vi "9235_9236_9237 4Ch Analog Input.vi"(1 "9235/9236/9237 I/O":T1={"9235/9236/9237 AI0"="NI 9235/AI0", "9235/9236/9237 AI1"="NI 9235/AI1", "9235/9236/9237 AI2"="NI 9235/AI2", "9235/9236/9237 AI3"="NI 9235/AI3"}) -> (0 "Packets":u64[](array[numeric]))   [LabVIEW 2010]
uses:
  <vilib>/eio/EIONode/EIONode.xnode
  <vilib>/rvi/eio/nirviEIOImplementation/nirviEIOImplementation.xnode
  <vilib>/rvi/eio/common/nirviEmuClasses.ctl
  <vilib>/rvi/eio/common/nirviEmuTemplateMethod_noerrors.vi
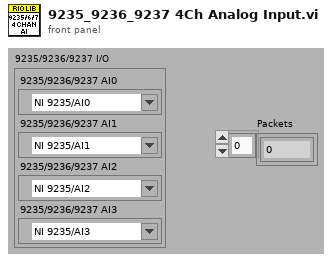
[diagram p1: front panel]
types:
  T1 = cluster{"9235/9236/9237 AI0":refnum<k21>, "9235/9236/9237 AI1":refnum<k21>, "9235/9236/9237 AI2":refnum<k21>, "9235/9236/9237 AI3":refnum<k21>}
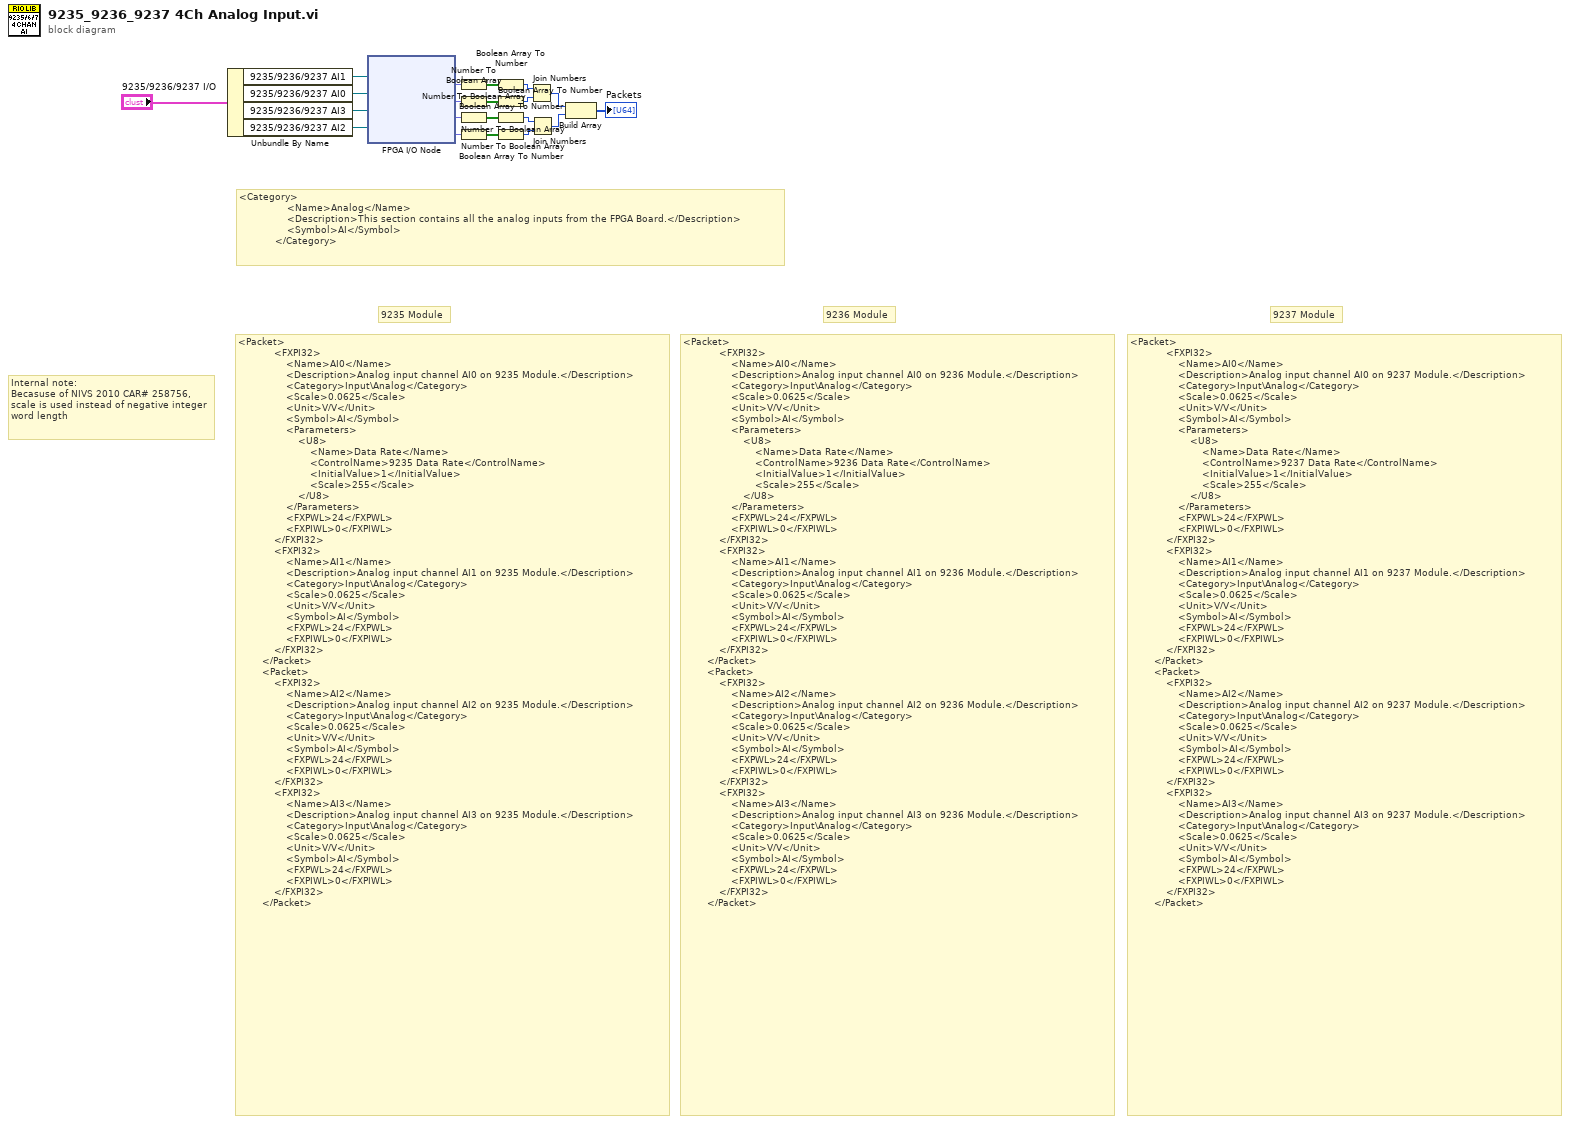
[diagram p0: block diagram]
diagram:
  # "9237 Module"
  # "<Packet>\n            <FXPI32>\n                <Name>AI0</Name>\n                <Description>Analog input channel AI0 on 9237 Module.</Description>\n                <Category>Input\\Analog</Category>\n                <Scale>0.0625</Scale>\n                <Unit>V/V</Unit>\n                <Symbol>AI</Symbol>\n                <Parameters>\n                    <U8>\n                        <Name>Data Rate</Name>\n                        <ControlName>9237 Data Rate</ControlName>\n                        <InitialValue>1</InitialValue>\n                        <Scale>255</Scale>\n                    </U8>\n                </Parameters>\n                <FXPWL>24</FXPWL>\n                <FXPIWL>0</FXPIWL>\n            </FXPI32>\n            <FXPI32>\n                <Name>AI1</Name>\n                <Description>Analog input channel AI1 on 9237 Module.</Description>\n                <Category>Input\\Analog</Category>\n                <Scale>0.0625</Scale>\n                <Unit>V/V</Unit>\n                <Symbol>AI</Symbol>\n                <FXPWL>24</FXPWL>\n                <FXPIWL>0</FXPIWL>\n            </FXPI32>\n        </Packet>\n        <Packet>\n            <FXPI32>\n                <Name>AI2</Name>\n                <Description>Analog input channel AI2 on 9237 Module.</Description>\n                <Category>Input\\Analog</Category>\n                <Scale>0.0625</Scale>\n                <Unit>V/V</Unit>\n                <Symbol>AI</Symbol>\n                <FXPWL>24</FXPWL>\n                <FXPIWL>0</FXPIWL>\n            </FXPI32>\n            <FXPI32>\n                <Name>AI3</Name>\n                <Description>Analog input channel AI3 on 9237 Module.</Description>\n                <Category>Input\\Analog</Category>\n                <Scale>0.0625</Scale>\n                <Unit>V/V</Unit>\n                <Symbol>AI</Symbol>\n                <FXPWL>24</FXPWL>\n                <FXPIWL>0</FXPIWL>\n            </FXPI32>\n        </Packet>"
  # "9236 Module"
  # "<Packet>\n            <FXPI32>\n                <Name>AI0</Name>\n                <Description>Analog input channel AI0 on 9236 Module.</Description>\n                <Category>Input\\Analog</Category>\n                <Scale>0.0625</Scale>\n                <Unit>V/V</Unit>\n                <Symbol>AI</Symbol>\n                <Parameters>\n                    <U8>\n                        <Name>Data Rate</Name>\n                        <ControlName>9236 Data Rate</ControlName>\n                        <InitialValue>1</InitialValue>\n                        <Scale>255</Scale>\n                    </U8>\n                </Parameters>\n                <FXPWL>24</FXPWL>\n                <FXPIWL>0</FXPIWL>\n            </FXPI32>\n            <FXPI32>\n                <Name>AI1</Name>\n                <Description>Analog input channel AI1 on 9236 Module.</Description>\n                <Category>Input\\Analog</Category>\n                <Scale>0.0625</Scale>\n                <Unit>V/V</Unit>\n                <Symbol>AI</Symbol>\n                <FXPWL>24</FXPWL>\n                <FXPIWL>0</FXPIWL>\n            </FXPI32>\n        </Packet>\n        <Packet>\n            <FXPI32>\n                <Name>AI2</Name>\n                <Description>Analog input channel AI2 on 9236 Module.</Description>\n                <Category>Input\\Analog</Category>\n                <Scale>0.0625</Scale>\n                <Unit>V/V</Unit>\n                <Symbol>AI</Symbol>\n                <FXPWL>24</FXPWL>\n                <FXPIWL>0</FXPIWL>\n            </FXPI32>\n            <FXPI32>\n                <Name>AI3</Name>\n                <Description>Analog input channel AI3 on 9236 Module.</Description>\n                <Category>Input\\Analog</Category>\n                <Scale>0.0625</Scale>\n                <Unit>V/V</Unit>\n                <Symbol>AI</Symbol>\n                <FXPWL>24</FXPWL>\n                <FXPIWL>0</FXPIWL>\n            </FXPI32>\n        </Packet>"
  # "Internal note:\nBecasuse of NIVS 2010 CAR# 258756, scale is used instead of negative integer word length"
  # "9235 Module"
  # "<Category>\n                <Name>Analog</Name>\n                <Description>This section contains all the analog inputs from the FPGA Board.</Description>\n                <Symbol>AI</Symbol>\n            </Category>"
  # "<Packet>\n            <FXPI32>\n                <Name>AI0</Name>\n                <Description>Analog input channel AI0 on 9235 Module.</Description>\n                <Category>Input\\Analog</Category>\n                <Scale>0.0625</Scale>\n                <Unit>V/V</Unit>\n                <Symbol>AI</Symbol>\n                <Parameters>\n                    <U8>\n                        <Name>Data Rate</Name>\n                        <ControlName>9235 Data Rate</ControlName>\n                        <InitialValue>1</InitialValue>\n                        <Scale>255</Scale>\n                    </U8>\n                </Parameters>\n                <FXPWL>24</FXPWL>\n                <FXPIWL>0</FXPIWL>\n            </FXPI32>\n            <FXPI32>\n                <Name>AI1</Name>\n                <Description>Analog input channel AI1 on 9235 Module.</Description>\n                <Category>Input\\Analog</Category>\n                <Scale>0.0625</Scale>\n                <Unit>V/V</Unit>\n                <Symbol>AI</Symbol>\n                <FXPWL>24</FXPWL>\n                <FXPIWL>0</FXPIWL>\n            </FXPI32>\n        </Packet>\n        <Packet>\n            <FXPI32>\n                <Name>AI2</Name>\n                <Description>Analog input channel AI2 on 9235 Module.</Description>\n                <Category>Input\\Analog</Category>\n                <Scale>0.0625</Scale>\n                <Unit>V/V</Unit>\n                <Symbol>AI</Symbol>\n                <FXPWL>24</FXPWL>\n                <FXPIWL>0</FXPIWL>\n            </FXPI32>\n            <FXPI32>\n                <Name>AI3</Name>\n                <Description>Analog input channel AI3 on 9235 Module.</Description>\n                <Category>Input\\Analog</Category>\n                <Scale>0.0625</Scale>\n                <Unit>V/V</Unit>\n                <Symbol>AI</Symbol>\n                <FXPWL>24</FXPWL>\n                <FXPIWL>0</FXPIWL>\n            </FXPI32>\n        </Packet>"
  n1 = Unbundle By Name("9235/9236/9237 I/O") -> ("9235/9236/9237 AI1"=w5:refnum<k21>, "9235/9236/9237 AI0"=w8:refnum<k21>, "9235/9236/9237 AI3"=w6:refnum<k21>, "9235/9236/9237 AI2"=w9:refnum<k21>)
  n2 = xnode "FPGA I/O Node"("FPGA I/O In"=w5, "FPGA I/O In"=w8, "FPGA I/O In"=w6, "FPGA I/O In"=w9) -> ("I/O Item"=w14:fxp<+/-,24,-4>, "I/O Item"=w16:fxp<+/-,24,-4>, "I/O Item"=w7:fxp<+/-,24,-4>, "I/O Item"=w15:fxp<+/-,24,-4>)  [unwired: 4 out]
  n3 = Number To Boolean Array(number=w14) -> (Boolean array=w10:bool[])
  n4 = Number To Boolean Array(number=w16) -> (Boolean array=w11:bool[])
  n5 = Number To Boolean Array(number=w7) -> (Boolean array=w13:bool[])
  n6 = Number To Boolean Array(number=w15) -> (Boolean array=w12:bool[])
  n7 = Boolean Array To Number(Boolean array=w10) -> (number=w17:u32)
  n8 = Boolean Array To Number(Boolean array=w11) -> (number=w18:u32)
  n9 = Boolean Array To Number(Boolean array=w13) -> (number=w19:u32)
  n10 = Boolean Array To Number(Boolean array=w12) -> (number=w20:u32)
  n11 = Join Numbers(hi=w17, lo=w18) -> ((hi.lo)=w3:u64)
  n12 = Join Numbers(hi=w19, lo=w20) -> ((hi.lo)=w4:u64)
  n13 = Build Array(w3, w4) -> (→"Packets":u64[])
